vi "Write last_error_test.vi"(10 "last_error":dbl, 11 "PIDController in":refnum<class "PIDController.lvclass">) -> (3 "PIDController out":refnum<class "PIDController.lvclass">)   [LabVIEW 2025, in "PIDController.lvclass"]
uses:
  PIDController.lvclass
  PIDController.lvclass/PIDController.ctl
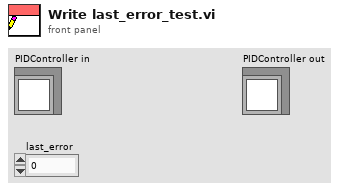
[diagram p1: front panel]
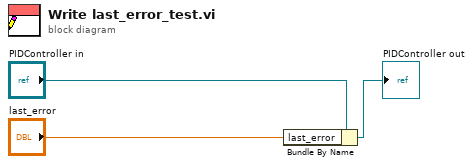
[diagram p0: block diagram]
diagram:
  n1 = Bundle By Name(cluster="PIDController in", "last_error"="last_error") -> (→"PIDController out":refnum<class "PIDController.lvclass">)
